vi "PPMS Interface_v230630.vi"() -> ()   [LabVIEW 2020]
panel:
  out "AC Flag":bool caption="AC Current"
  in  "Filetype":u16(ring)=2 items=[".xlsx", ".txt", ".csv"]
  out "Wait Done":dbl=10.0
  in  "Measurement setup tabs":enum32{"DC Setup", "AC Setup", "DC Delta Mode"}(tab)=enum."AC Setup"
  in  "DC Pulse":bool=TRUE caption="Current Pulsing"
  in  "Channel 2":bool=TRUE
  in  "Channel 1":bool
  in  "Current Amplitude":string="5e-4"
  in  "Time Period (s)":string="3"
  in  "Tpad(ms)":i32=200
  in  "Voltmeter Range (V)":string="0.01"
  in  "NPLC":string="1"
  in  "Voltmeter Buffer Size":string="62"
  in  "Voltmeter 2 Address":string="7"
  in  "Voltmeter 1 Address":string="8"
  in  "6221 Address":string="12"
  in  "Configure DC System":bool
  in  "6221 Address 2":string="12" caption="6221 Address"
  in  "Current Amplitude 2":string="100e-6" caption="Current \nAmplitude"
  in  "Ch2 Enable":bool=TRUE
  in  "Ch1 Enable":bool=TRUE
  in  "Buffer Data":enum16{"X", "XY", "RT", "XYRT"}(ring)=enum."RT"
  in  "Rate decimation":i32=2
  in  "SR860 Ch2 Address":string="5"
  in  "SR860 Ch1 Address":string="4"
  in  "Frequency":string="1711"
  in  "Filter BW":T1(ring)=enum."100ms"
  in  "Ch1 Harmonic":T2(ring)
  in  "Buffer Size (kB)":i32=2
  in  "Configure AC System":bool
  in  "Buffer Offset (kb)":string="0"
  in  "Ch2 Harmonic":T2(ring)=enum."2nd Harmonic"
  in  "Measurement \nSetup":u16(ring) items=["DC Setup", "AC Setup", "DC Delta Mode"]
  in  "Measure Device":bool caption="Measure \nDevice"
  in  "Y-axis":u16(ring)=6 items=["Serial Number", "Time Elapsed (s)", "Temperature (K)", "Field (Oe)", "Theta (degree)", "Current excitation (A)", "Resistance 1 (ohm)", "STD 1 (ohm)", "Resistance 2 (ohm)", "STD 2 (ohm)"]
  in  "X-axis":u16(ring)=3 items=["Serial Number", "Time Elapsed (s)", "Temperature (K)", "Field (Oe)", "Theta (degree)", "Current excitation (A)", "Resistance 1 (ohm)", "STD 1 (ohm)", "Resistance 2 (ohm)", "STD 2 (ohm)"]
  out "XY Graph":cluster{"Data array":dbl[], "Data array":dbl[]}(graph)={"Data array"=[1000.1076049804688, 1000.095458984375, 1000.1318969726562, 999.822021484375, 916.6700439453125, 830.8634643554688, 742.8192749023438, 654.9420776367188, 567.0899047851562, 479.1545104980469, 392.864013671875, 304.93212890625, 216.95523071289062, 129.0848846435547, 41.132198333740234, -44.77364730834961, -132.77415466308594, -218.81509399414062, -306.63739013671875, -394.50677490234375, -482.4195251464844, -570.4457397460938, -658.3638305664062, -744.2162475585938, -832.0615234375, -920.28857421875, -999.9136352539062, -999.8893432617188, -999.877197265625, -966.5936279296875, -880.3653564453125, -790.4647827148438, -704.466064453125, -616.628173828125, -528.7174682617188, -442.6363525390625, -352.7901916503906, -266.7317810058594, -178.9671173095703, -91.0753402709961, -3.042452096939087, 84.87220001220703, 170.94114685058594, 258.7779235839844, 346.6785583496094, 434.949462890625, 520.9051513671875, 608.9139404296875, 696.776611328125, 782.679931640625, 870.5813598632812, 958.4483642578125, 1000.1197509765625, 1000.095458984375], "Data array"=[2.0974435134090905, 2.0958316086363635, 2.0992071125, 2.0990977595454545, 2.107740888863636, 2.1053484827272726, 2.1082263649999997, 2.1037182222727275, 2.083242016590909, 2.081601890227273, 2.0829138438636363, 2.0798880874999996, 2.0791002761363635, 2.0677500127272728, 1.8619974204545455, 1.1222847387045454, 0.8201078938409091, 0.7255154414090907, 0.6976336516363636, 0.7003691852045455, 0.6927557248181818, 0.7014058921818181, 0.6990065759090907, 0.7079667083181819, 0.7010926857727272, 0.6957325292954544, 0.6955325533636365, 0.697872530181818, 0.711508848840909, 0.7229268473181818, 0.7067185125454545, 0.6959014081136364, 0.6962725788181818, 0.7031570712499998, 0.6892584726363638, 0.6798120112272727, 0.6948854190227274, 0.70866324875, 0.7220332009318181, 0.7281562234318182, 1.006325211, 1.7135642684090908, 1.949954792045455, 2.0590681531818182, 2.084260665, 2.087814913863636, 2.0882882709090906, 2.090093333181818, 2.0964560554545457, 2.1017757368181815, 2.103902046363636, 2.0958079104545453, 2.1060686974999996, 2.0965902061363635]}
  out "WAIT delay(s)":u32=10
  out "Data array":dbl[][](array[numeric])=[[1.0, 4.4622015953063965, 299.982421875, 1000.1076049804688, -0.00037384033203125, 0.0001, 2.0974435134090905, 0.003970427238917819, 0.023133111600000002, 0.00015789614384998], [2.0, 8.857791900634766, 299.9828186035156, 1000.095458984375, -0.00037384033203125, 0.0001, 2.0958316086363635, 0.005717710280839478, 0.023133111600000002, 0.00015789614384998], [3.0, 13.236927509307861, 299.9828186035156, 1000.1318969726562, -0.00037384033203125, 0.0001, 2.0992071125, 0.006189541986117072, 0.023133111600000002, 0.00015789614384998], [4.0, 17.593226432800293, 299.98480224609375, 999.822021484375, -0.00037384033203125, 0.0001, 2.0990977595454545, 0.003912224013200419, 0.023133111600000002, 0.00015789614384998], [5.0, 21.948697090148926, 299.9840087890625, 916.6700439453125, -0.00037384033203125, 0.0001, 2.107740888863636, 0.005090003201604339, 0.023133111600000002, 0.00015789614384998], [6.0, 26.332980155944824, 299.98516845703125, 830.8634643554688, -0.00037384033203125, 0.0001, 2.1053484827272726, 0.005739735103255567, 0.023133111600000002, 0.00015789614384998], [7.0, 30.68852186203003, 299.985595703125, 742.8192749023438, -0.00037384033203125, 0.0001, 2.1082263649999997, 0.005571697815375255, 0.023133111600000002, 0.00015789614384998], [8.0, 35.09347057342529, 299.98638916015625, 654.9420776367188, -0.00037384033203125, 0.0001, 2.1037182222727275, 0.00788260633201801, 0.023133111600000002, 0.00015789614384998], [9.0, 39.4463529586792, 299.98480224609375, 567.0899047851562, -0.00037384033203125, 0.0001, 2.083242016590909, 0.006414237562318937, 0.023133111600000002, 0.00015789614384998], [10.0, 43.830984115600586, 299.9861755371094, 479.1545104980469, -0.00037384033203125, 0.0001, 2.081601890227273, 0.005074439315863804, 0.023133111600000002, 0.00015789614384998], [11.0, 48.21513843536377, 299.98516845703125, 392.864013671875, -0.00037384033203125, 0.0001, 2.0829138438636363, 0.0047092558667783495, 0.023133111600000002, 0.00015789614384998], [12.0, 52.58274984359741, 299.9877624511719, 304.93212890625, -0.00037384033203125, 0.0001, 2.0798880874999996, 0.007156650519378263, 0.023133111600000002, 0.00015789614384998], [13.0, 56.942962646484375, 299.9867858886719, 216.95523071289062, -0.00037384033203125, 0.0001, 2.0791002761363635, 0.006338073258755396, 0.023133111600000002, 0.00015789614384998], [14.0, 61.33445596694946, 299.9844055175781, 129.0848846435547, -0.00037384033203125, 0.0001, 2.0677500127272728, 0.004479419760797201, 0.023133111600000002, 0.00015789614384998], [15.0, 65.69865989685059, 299.98516845703125, 41.132198333740234, -0.00037384033203125, 0.0001, 1.8619974204545455, 0.04372637509011968, 0.023133111600000002, 0.00015789614384998], [16.0, 70.06871700286865, 299.985595703125, -44.77364730834961, -0.00037384033203125, 0.0001, 1.1222847387045454, 0.04141744482498131, 0.023133111600000002, 0.00015789614384998], [17.0, 74.4264874458313, 299.98516845703125, -132.77415466308594, -0.00037384033203125, 0.0001, 0.8201078938409091, 0.012918566246848149, 0.023133111600000002, 0.00015789614384998], [18.0, 78.80255699157715, 299.985595703125, -218.81509399414062, -0.00037384033203125, 0.0001, 0.7255154414090907, 0.013867678751370198, 0.023133111600000002, 0.00015789614384998], [19.0, 83.20550107955933, 299.985595703125, -306.63739013671875, -0.00037384033203125, 0.0001, 0.6976336516363636, 0.005727042126808915, 0.023133111600000002, 0.00015789614384998], [20.0, 87.57900810241699, 299.9859619140625, -394.50677490234375, -0.00037384033203125, 0.0001, 0.7003691852045455, 0.006164392957730509, 0.023133111600000002, 0.00015789614384998], [21.0, 91.95004034042358, 299.98577880859375, -482.4195251464844, -0.00037384033203125, 0.0001, 0.6927557248181818, 0.005210320909525348, 0.023133111600000002, 0.00015789614384998], [22.0, 96.33998107910156, 299.9861755371094, -570.4457397460938, -0.00037384033203125, 0.0001, 0.7014058921818181, 0.004608349946130019, 0.023133111600000002, 0.00015789614384998], [23.0, 100.71973752975464, 299.98577880859375, -658.3638305664062, -0.00037384033203125, 0.0001, 0.6990065759090907, 0.003365288674988466, 0.023133111600000002, 0.00015789614384998], [24.0, 105.0504822731018, 299.98638916015625, -744.2162475585938, -0.00037384033203125, 0.0001, 0.7079667083181819, 0.006059950157953656, 0.023133111600000002, 0.00015789614384998], [25.0, 109.43017148971558, 299.9879455566406, -832.0615234375, -0.00037384033203125, 0.0001, 0.7010926857727272, 0.006067166646240939, 0.023133111600000002, 0.00015789614384998], [26.0, 113.79940557479858, 299.9875793457031, -920.28857421875, -0.00037384033203125, 0.0001, 0.6957325292954544, 0.005627155853698697, 0.023133111600000002, 0.00015789614384998], [27.0, 118.25392484664917, 299.9867858886719, -999.9136352539062, -0.00037384033203125, 0.0001, 0.6955325533636365, 0.00707814850177566, 0.023133111600000002, 0.00015789614384998], [28.0, 122.64683437347412, 299.985595703125, -999.8893432617188, -0.00037384033203125, 0.0001, 0.697872530181818, 0.004908374987900224, 0.023133111600000002, 0.00015789614384998], [29.0, 127.02530670166016, 299.9861755371094, -999.877197265625, -0.00037384033203125, 0.0001, 0.711508848840909, 0.004892085657814586, 0.023133111600000002, 0.00015789614384998], [30.0, 131.39422178268433, 299.98516845703125, -966.5936279296875, -0.00037384033203125, 0.0001, 0.7229268473181818, 0.0044813852811875655, 0.023133111600000002, 0.00015789614384998], [31.0, 135.83348321914673, 299.9867858886719, -880.3653564453125, -0.00037384033203125, 0.0001, 0.7067185125454545, 0.004279656852638706, 0.023133111600000002, 0.00015789614384998], [32.0, 140.21209907531738, 299.98516845703125, -790.4647827148438, -0.00037384033203125, 0.0001, 0.6959014081136364, 0.005017213765156999, 0.023133111600000002, 0.00015789614384998], [33.0, 144.59554243087769, 299.98638916015625, -704.466064453125, -0.00037384033203125, 0.0001, 0.6962725788181818, 0.007024556533565583, 0.023133111600000002, 0.00015789614384998], [34.0, 148.9465184211731, 299.9861755371094, -616.628173828125, -0.00037384033203125, 0.0001, 0.7031570712499998, 0.006011419658937474, 0.023133111600000002, 0.00015789614384998], [35.0, 153.31742238998413, 299.9883728027344, -528.7174682617188, -0.00037384033203125, 0.0001, 0.6892584726363638, 0.0056657125166453695, 0.023133111600000002, 0.00015789614384998], [36.0, 157.72580194473267, 299.9879455566406, -442.6363525390625, -0.00037384033203125, 0.0001, 0.6798120112272727, 0.006911608247074455, 0.023133111600000002, 0.00015789614384998], [37.0, 162.09323120117188, 299.98895263671875, -352.7901916503906, -0.00037384033203125, 0.0001, 0.6948854190227274, 0.005234077839025774, 0.023133111600000002, 0.00015789614384998], [38.0, 166.4765763282776, 299.9881591796875, -266.7317810058594, -0.00037384033203125, 0.0001, 0.70866324875, 0.004897465156522533, 0.023133111600000002, 0.00015789614384998], [39.0, 170.89887046813965, 299.9877624511719, -178.9671173095703, -0.00037384033203125, 0.0001, 0.7220332009318181, 0.004374043049098589, 0.023133111600000002, 0.00015789614384998], [40.0, 175.30081844329834, 299.98895263671875, -91.0753402709961, -0.00037384033203125, 0.0001, 0.7281562234318182, 0.004378933623760837, 0.023133111600000002, 0.00015789614384998], [41.0, 179.67326831817627, 299.9881591796875, -3.042452096939087, -0.00037384033203125, 0.0001, 1.006325211, 0.05479208135231416, 0.023133111600000002, 0.00015789614384998], [42.0, 184.02438020706177, 299.9891662597656, 84.87220001220703, -0.00037384033203125, 0.0001, 1.7135642684090908, 0.031492821331516825, 0.023133111600000002, 0.00015789614384998], [43.0, 188.40718173980713, 299.9934997558594, 170.94114685058594, -0.00037384033203125, 0.0001, 1.949954792045455, 0.005867722136927017, 0.023133111600000002, 0.00015789614384998], [44.0, 192.7843451499939, 299.992919921875, 258.7779235839844, -0.00037384033203125, 0.0001, 2.0590681531818182, 0.005339923736116385, 0.023133111600000002, 0.00015789614384998], [45.0, 197.14294481277466, 299.9942932128906, 346.6785583496094, -0.00037384033203125, 0.0001, 2.084260665, 0.006323898951825988, 0.023133111600000002, 0.00015789614384998], [46.0, 201.48842906951904, 299.9949035644531, 434.949462890625, -0.00037384033203125, 0.0001, 2.087814913863636, 0.005555079114947601, 0.023133111600000002, 0.00015789614384998], [47.0, 205.88358163833618, 299.9934997558594, 520.9051513671875, -0.00037384033203125, 0.0001, 2.0882882709090906, 0.006813247199825648, 0.023133111600000002, 0.00015789614384998], [48.0, 210.2482304573059, 299.9954833984375, 608.9139404296875, -0.00037384033203125, 0.0001, 2.090093333181818, 0.004951890810177865, 0.023133111600000002, 0.00015789614384998], [49.0, 214.59800720214844, 299.9941101074219, 696.776611328125, -0.00037384033203125, 0.0001, 2.0964560554545457, 0.005307616082520529, 0.023133111600000002, 0.00015789614384998], [50.0, 218.96898794174194, 299.99371337890625, 782.679931640625, -0.00037384033203125, 0.0001, 2.1017757368181815, 0.004526206790352821, 0.023133111600000002, 0.00015789614384998], [51.0, 223.39048957824707, 299.9945068359375, 870.5813598632812, -0.00037384033203125, 0.0001, 2.103902046363636, 0.005438989400576699, 0.023133111600000002, 0.00015789614384998], [52.0, 227.7996335029602, 299.99609375, 958.4483642578125, -0.00037384033203125, 0.0001, 2.0958079104545453, 0.005075665798007201, 0.023133111600000002, 0.00015789614384998], [53.0, 232.15194511413574, 299.9954833984375, 1000.1197509765625, -0.00037384033203125, 0.0001, 2.1060686974999996, 0.004951135996534981, 0.023133111600000002, 0.00015789614384998], [54.0, 236.54437589645386, 299.9950866699219, 1000.095458984375, -0.00037384033203125, 0.0001, 2.0965902061363635, 0.00573349701852997, 0.023133111600000002, 0.00015789614384998]]
  out "Time Elasped":dbl format="%#_13g"
  out "Serial Number":i32=55
  out "Current StartTime":timestamp=timestamp(3772308572.9414487 s since 1904-01-01)
  out "Current Filename":path=path "C:/Users/qmgmit/Desktop/Shivam/data/FGaT-WTe2/20230715_FGaT-WTe2_chip3_D1/test_sweep_0715_1929.csv"
  in  "Metadata":string="NbSe2 C1 6L\n50 uA, Rxx on Ch 2\n"
  out "SET Rate":dbl=20.0
  out "SET Setpoint":dbl=1000.0
  out "Current Line Number":i32=10
  out "Parameters":dbl[][](array[numeric])
  out "ENV VAR":string="MEASURE"
  out "Current Line":string="STOP MEASURE "
  out "Command":string="STOP"
  in  "Datafile Path":path=path "C:/Users/QDUser/Desktop/User Data/Shivam/NbSe2 devices/C1_6L/cooldown"
  out "Line Count":i32=10
  out "Array of commands":string[][](array[string])=[["## Field sweep to test device health"], ["NEWFILE test_sweep"], [""], ["START MEASURE"], ["WAIT MEASURE 10"], ["SET FIELD -1000 RATE 20"], ["WAIT FIELD 10"], ["SET FIELD 1000 RATE 20"], ["WAIT FIELD 10"], ["STOP MEASURE "]]
  out "Sequence File":string="## Field sweep to test device health\nNEWFILE test_sweep\n\nSTART MEASURE\nWAIT MEASURE 10\nSET FIELD -1000 RATE 20\nWAIT FIELD 10\nSET FIELD 1000 RATE 20\nWAIT FIELD 10\nSTOP MEASURE "
  in  "Sequence File":path=path "C:/Users/QDUser/Desktop/User Data/Shivam/NbSe2 devices/C1_6L/cooldown.lseq"
  out "STOP Flag":bool=TRUE
  out "Measure Blink":bool
  in  "Stop sequence":bool
  in  "Start Sequence":bool caption="Set Temperature"
  out "ExecSeq":bool caption="Executing Sequence"
  out "Measure Flag":bool caption="Measurement in progress"
  out "Field\nStatus":i32(ring)=4 items=["MagnetUnknown"=0, "StablePersistent"=1, "WarmingSwitch"=2, "CoolingSwitch"=3, "StableDriven"=4, "Iterating"=5, "Charging"=6, "Discharging"=7, "CurrentError"=8, "MagnetFailure"=15]
  out "Temperature\nStatus":i32(ring)=1 items=["TemperatureUnknown"=0, "Stable"=1, "Tracking"=2, "Near"=5, "Chasing"=6, "Filling"=7, "Standby"=10, "Disabled"=13, "ImpedanceNotFunction"=14, "TempFailure"=15]
  out "Chamber\nStatus":i32(ring)=1 items=["ChamberUnknown"=0, "PurgedAndSealed"=1, "VentedAndSealed"=2, "Sealed"=3, "Purging"=4, "Venting"=5, "PreHiVac"=6, "HighVac"=7, "PumpContinuous"=8, "VentContinuous"=9, "ChamberFailure"=15]
  out "Initialised":bool=TRUE
  in  "STOP Button":bool=TRUE
  in  "Set Chamber":bool caption="Set Temperature"
  in  "Set Position":bool caption="Set Temperature"
  in  "Set Field":bool caption="Set Temperature"
  in  "Set Temperature":bool
  in  "Chamber Setpoint":i32(ring)=5 caption="Chamber" items=["Seal", "PurgeAndSeal", "VentAndSeal", "PumpContinuous", "VentContinuous", "HighVacuum"]
  out "Theta":dbl=-0.00017547607421875 caption="Position"
  in  "Theta Setpoint":dbl caption="Theta (degrees)" min=-10.0 max=370.0
  out "Field":dbl=0.03621025010943413
  out "Temperature":dbl=299.9980773925781
  in  "Field Setpoint":dbl caption="Field (Oe)" min=-90000.0 max=90000.0
  in  "Temperature setpoint":dbl=10.0 caption="Temperature (K)" min=1.8 max=400.0
  in  "InstrumentType":i32(ring)=2 items=["PPMS", "VersaLab", "DynaCool", "SVSM", "OptiCool"]
  in  "Remote \nMode":bool
  in  "IP Address":string="10.29.163.8"
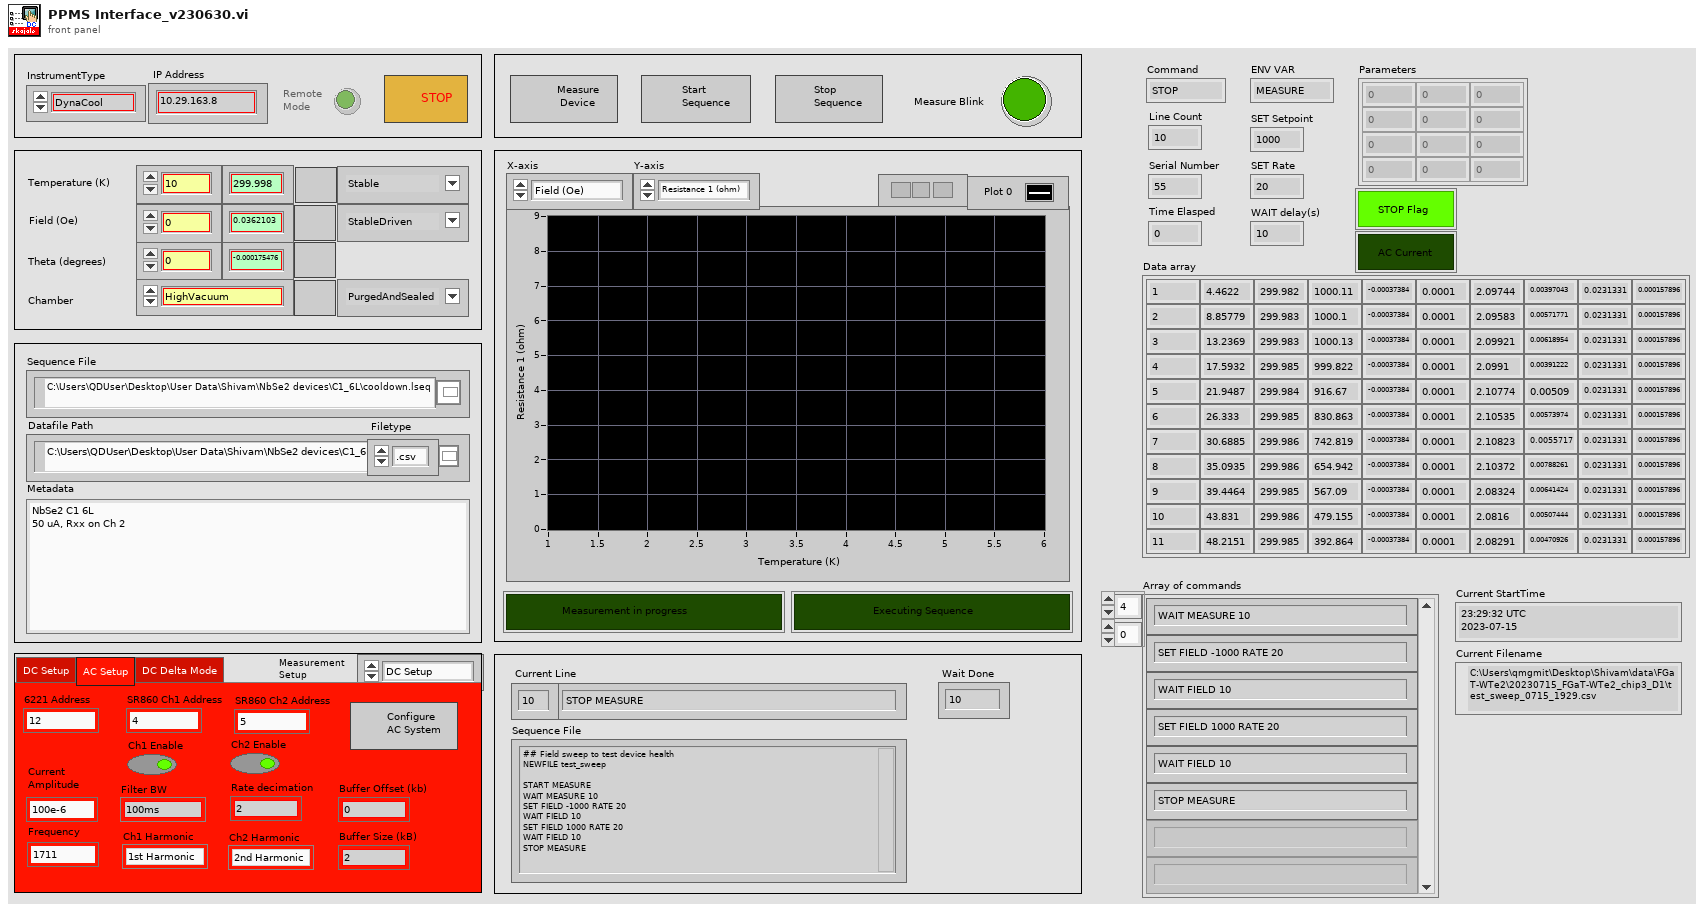
[diagram p1: front panel]
types:
  T1 = enum16{"1us", "3us", "10us", "30us", "100us", "300us", "1ms", "3ms", "10ms", "30ms", "100ms", "300ms", "1s"}
  T2 = enum16{"1st Harmonic", "2nd Harmonic", "3rd Harmonic"}
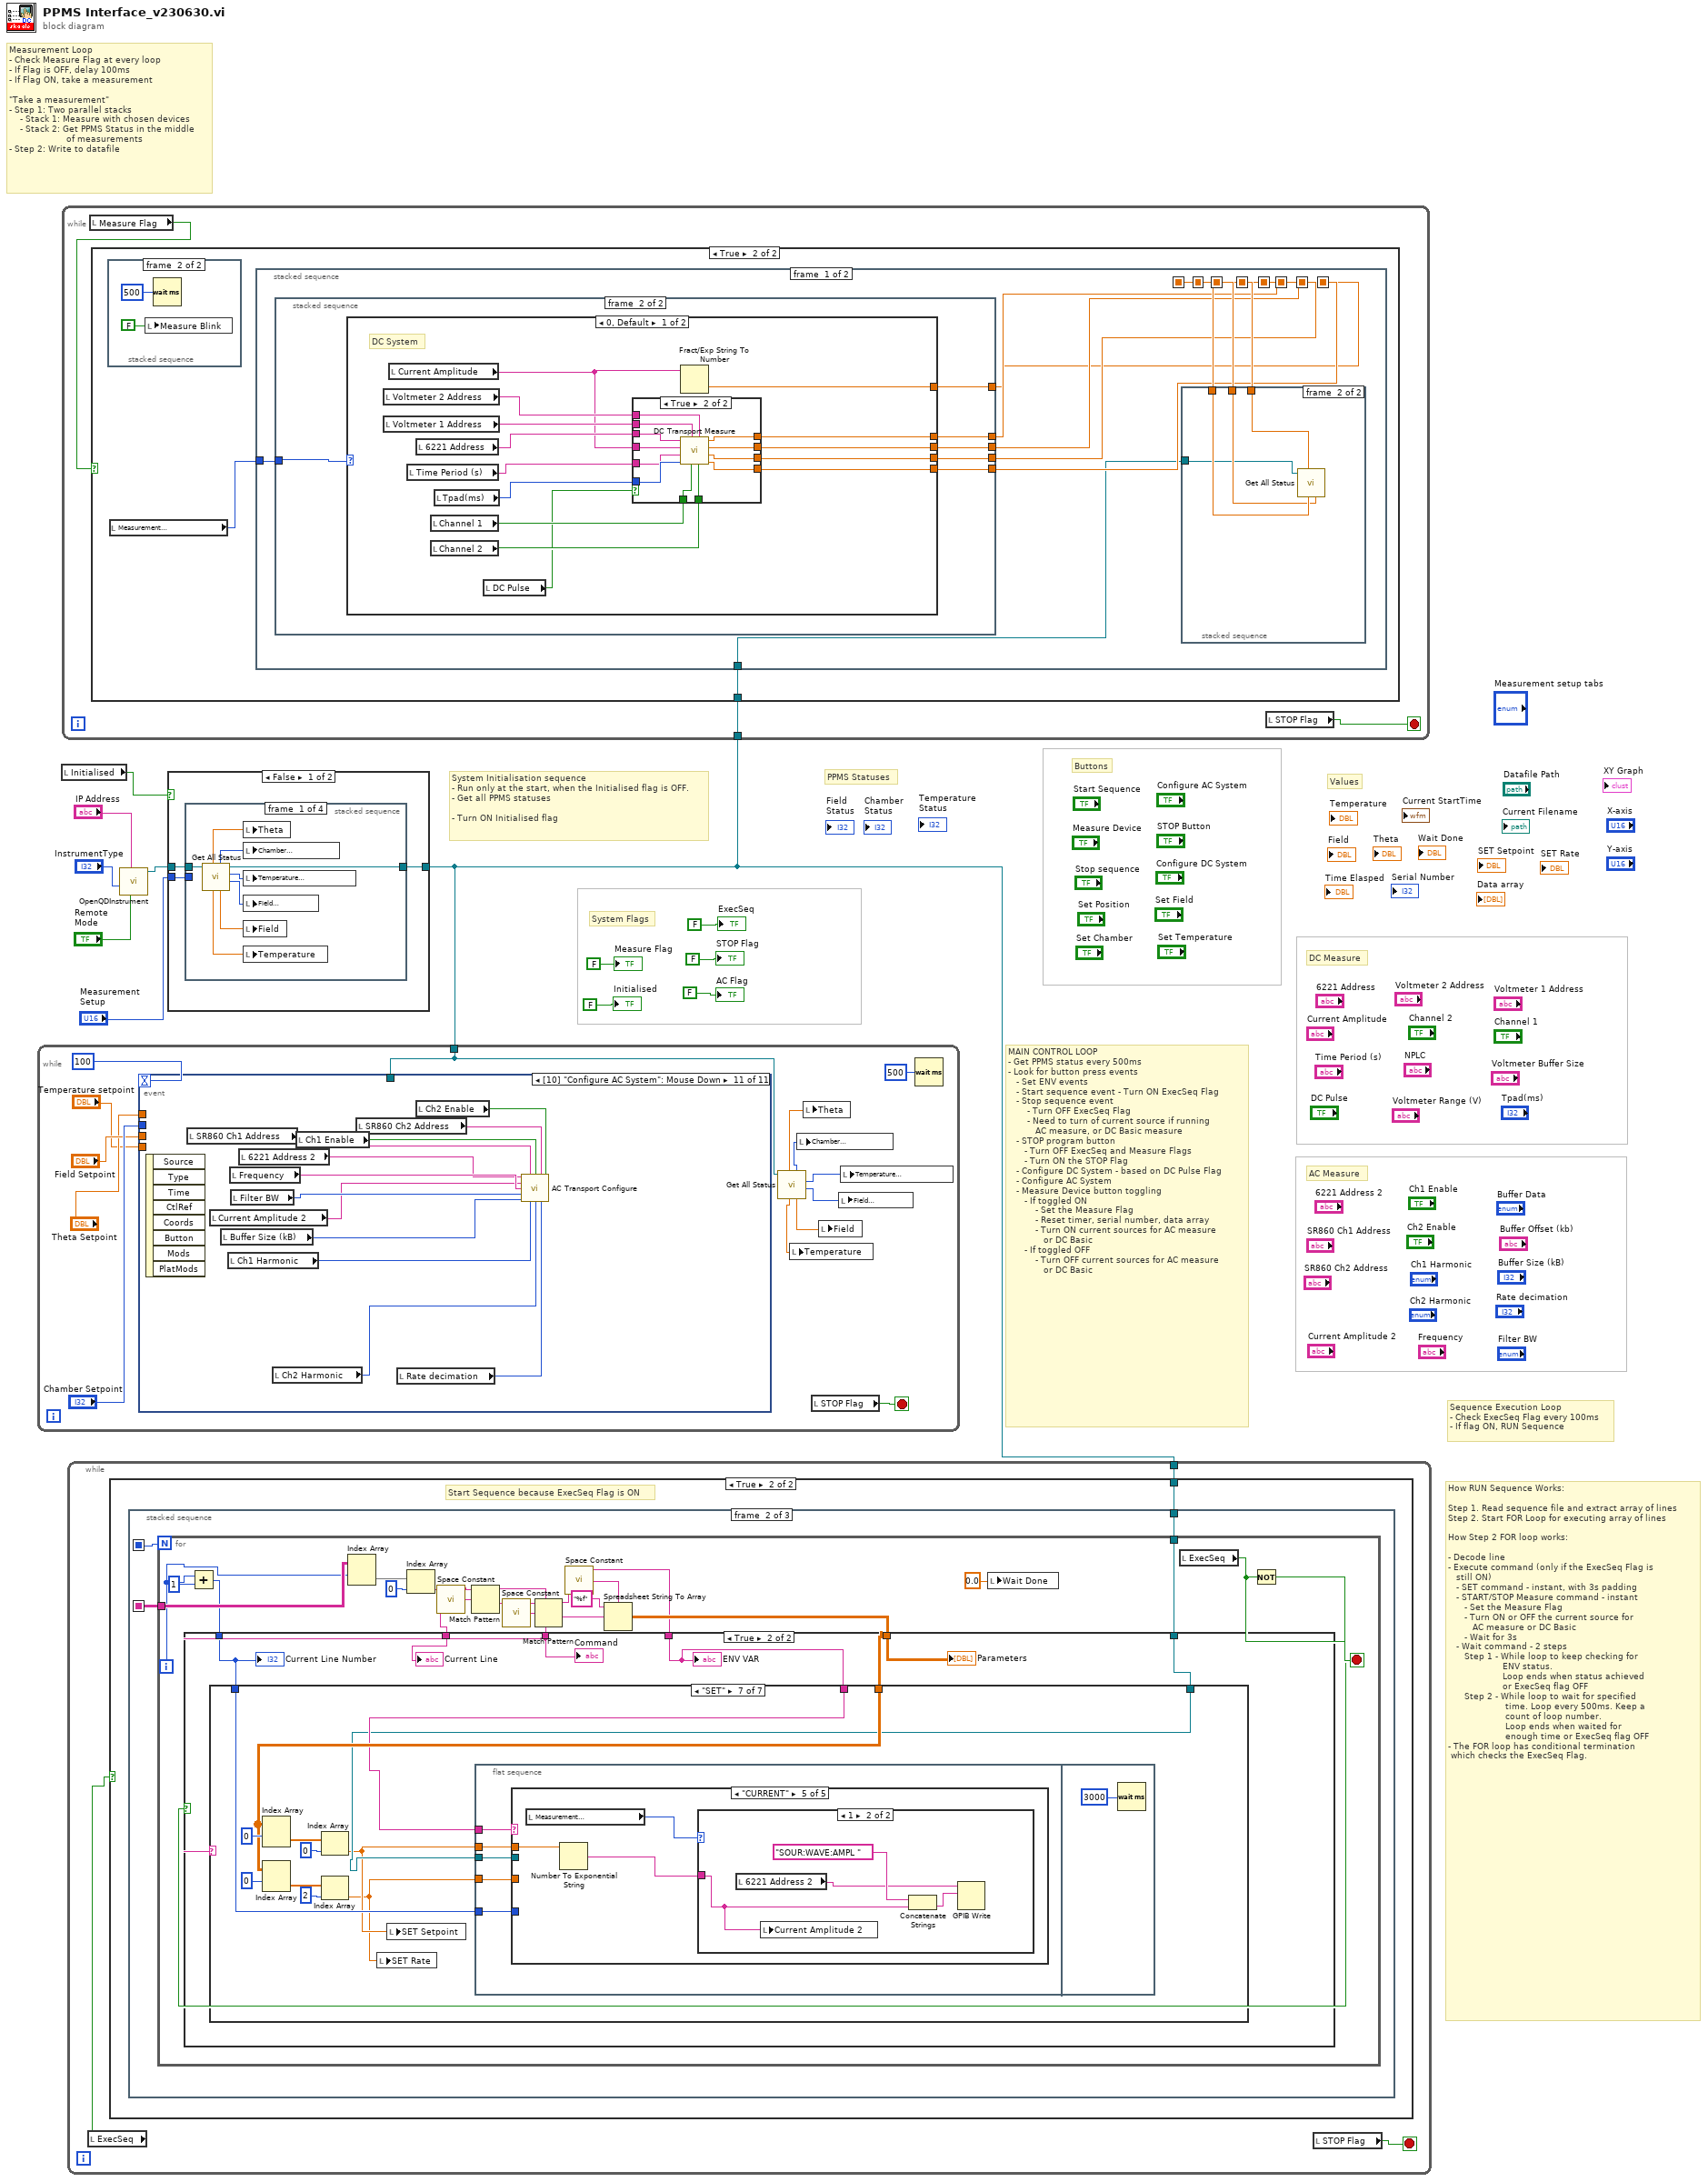
[diagram p0: block diagram]
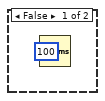
[diagram p2: hidden frame]
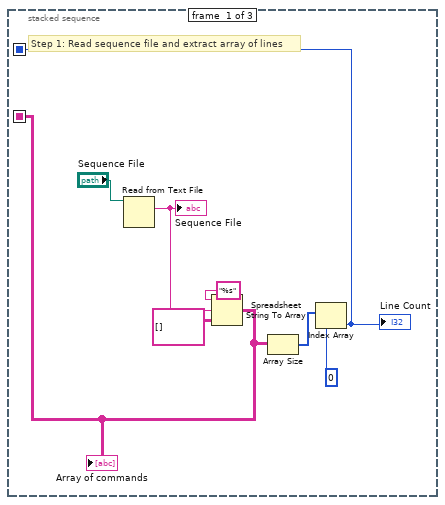
[diagram p3: hidden frame]
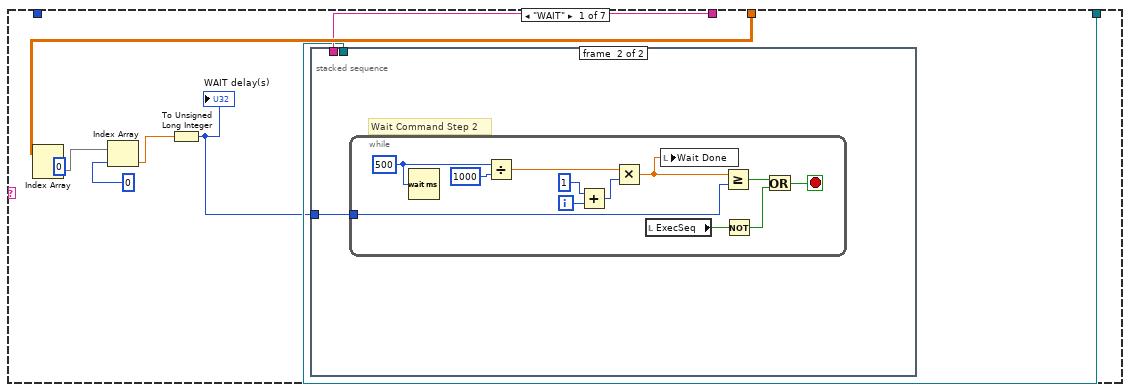
[diagram p5: hidden frame]
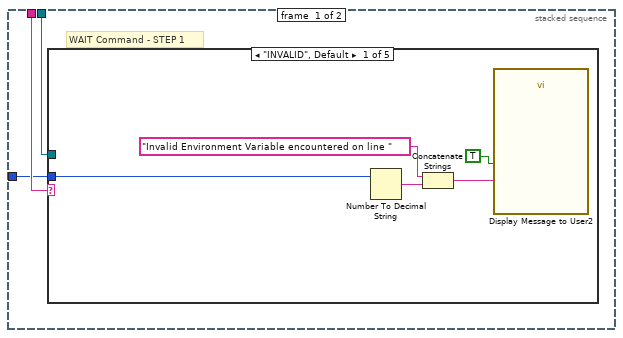
[diagram p6: hidden frame]
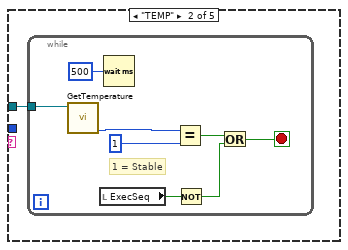
[diagram p7: hidden frame]
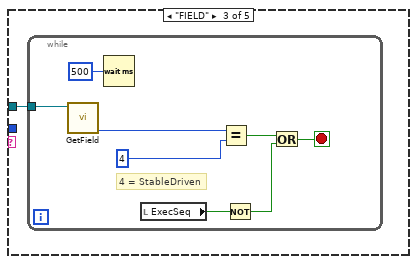
[diagram p8: hidden frame]
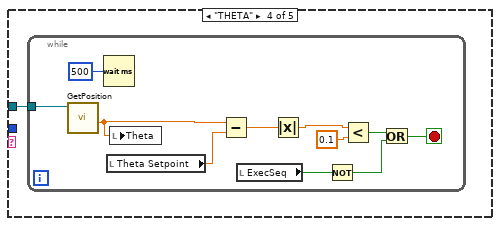
[diagram p9: hidden frame]
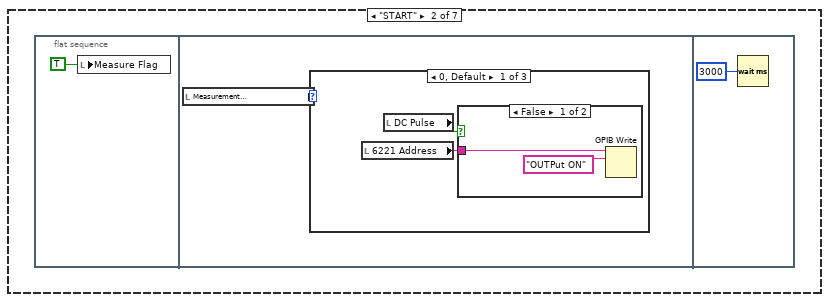
[diagram p11: hidden frame]
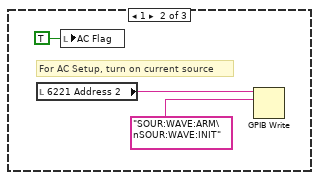
[diagram p13: hidden frame]
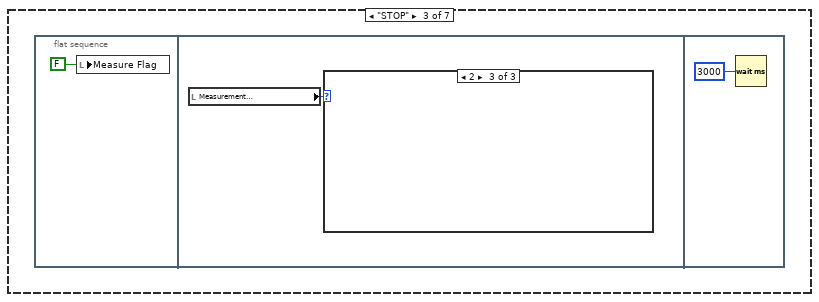
[diagram p15: hidden frame]
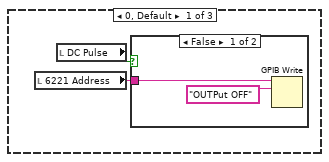
[diagram p16: hidden frame]
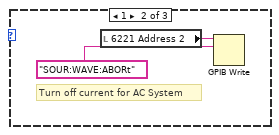
[diagram p18: hidden frame]
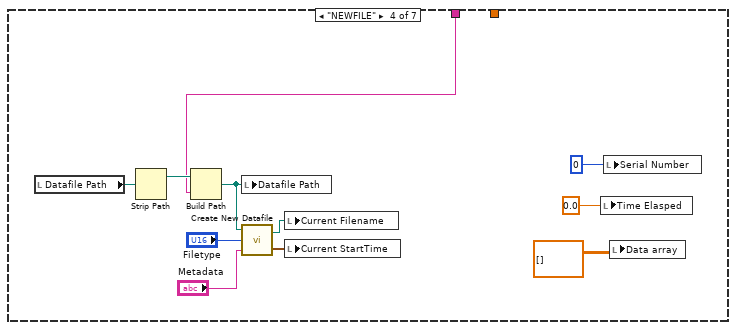
[diagram p19: hidden frame]
diagram:
  # "AC Measure"
  # "DC Measure"
  # "How RUN Sequence Works:\n\nStep 1. Read sequence file and extract array of lines \nStep 2. Start FOR Loop for executing array of lines\n\nHow Step 2 FOR loop works:\n\n- Decode line\n- Execute command (only if the ExecSeq Flag is \n   still ON)\n   - SET command - instant, with 3s padding\n   - START/STOP Measure command - instant\n      - Set the Measure Flag\n      - Turn ON or OFF the current source for \n         AC measure or DC Basic\n      - Wait for 3s\n   - Wait command - 2 steps\n      Step 1 - While loop to keep checking for\n                    ENV status.\n                    Loop ends when status achieved \n                    or ExecSeq flag OFF\n      Step 2 - While loop to wait for specified \n                     time. Loop every 500ms. Keep a \n                     count of loop number.\n                     Loop ends when waited for \n                     enough time or ExecSeq flag OFF\n- The FOR loop has conditional termination\n which checks the ExecSeq Flag."
  # "Sequence Execution Loop\n- Check ExecSeq Flag every 100ms\n- If flag ON, RUN Sequence"
  # "MAIN CONTROL LOOP\n- Get PPMS status every 500ms\n- Look for button press events\n   - Set ENV events\n   - Start sequence event - Turn ON ExecSeq Flag\n   - Stop sequence event \n       - Turn OFF ExecSeq Flag\n       - Need to turn of current source if running\n          AC measure, or DC Basic measure\n   - STOP program button \n      - Turn OFF ExecSeq and Measure Flags\n      - Turn ON the STOP Flag\n   - Configure DC System - based on DC Pulse Flag\n   - Configure AC System\n   - Measure Device button toggling\n      - If toggled ON \n          - Set the Measure Flag\n          - Reset timer, serial number, data array\n          - Turn ON current sources for AC measure \n             or DC Basic\n      - If toggled OFF\n          - Turn OFF current sources for AC measure \n             or DC Basic"
  # "System Flags"
  # "PPMS Statuses"
  # "Values"
  # "Buttons"
  # "System Initialisation sequence\n- Run only at the start, when the Initialised flag is OFF.\n- Get all PPMS statuses\n\n- Turn ON Initialised flag"
  # "Measurement Loop\n- Check Measure Flag at every loop\n- If Flag is OFF, delay 100ms\n- If Flag ON, take a measurement\n\n\"Take a measurement\"\n- Step 1: Two parallel stacks\n    - Stack 1: Measure with chosen devices\n    - Stack 2: Get PPMS Status in the middle\n                     of measurements\n- Step 2: Write to datafile"
  n1 = local read "Initialised"() -> (w8:bool)
  n2 = call "OpenQDInstrument.vi"("Remote"="Remote \nMode", "IP Address"="IP Address", "InstrumentType"="InstrumentType") -> ("Instrument Ref"=w7:refnum<k24>)  [unwired: 5 in, 1 out]
  n3 = case shown="False" w8 {
    tunnel: w7 -> [w15 w26]
    tunnel: [w14 w26] -> w3
    tunnel: "Measurement \nSetup" -> [w13 _]
    frame False {
      n4 = stacked-sequence {
        tunnel: w15 -> [w23 _ _ _]
        tunnel: [w17 _ _ _] -> w14
        tunnel: w13 -> [_ _ _ _]
        frame #0 {
          n5 = call "Get All Status.vi"("Instrument Ref In"=w23) -> ("Field\nStatus"=w20:i32, "Temperature\nStatus"=w21:i32, "Instrument Ref Out"=w17:refnum<k24>, "Field"=w18:dbl, "Chamber\nStatus"=w22:i32, "Temperature"=w19:dbl, "Position"=w16:dbl)  [unwired: 3 in, 1 out]
          n6 = local write "Theta"(w16) -> ()
          n7 = local write "Chamber\nStatus"(w22) -> ()
          n8 = local write "Temperature\nStatus"(w21) -> ()
          n9 = local write "Field\nStatus"(w20) -> ()
          n10 = local write "Field"(w18) -> ()
          n11 = local write "Temperature"(w19) -> ()
        }
        frame #1 {
          n12 = Wait (ms)(milliseconds to wait=u32 100) -> ()  [unwired: 1 out]
        }
        frame #2 {
        }
        frame #3 {
          n13 = local write "Initialised"(TRUE ("Initialised")) -> ()
        }
      }
    }
    frame True {
    }
  }
  n14 = while {
    tunnel: w3 -> [w31]
    stop <- w28 stop-if-true
    n15 = event shown="[10] \"Configure AC System\": Mouse Down" {
      selector: _ -> [_ _ _ _ _ _ _ _ _ _ _]
      dyn-events: _ -> [_ _ _ _ _ _ _ _ _ _ _]
      timeout: 100 -> [_ _ _ _ _ _ _ _ _ _ _]
      tunnel: "Chamber Setpoint" -> [_ _ w72 _ _ _ _ _ _ _ _]
      tunnel: w31 -> [_ _ w71 w76 w78 w82 _ _ _ _ _]
      tunnel: "Temperature setpoint" -> [_ _ _ w73 _ _ _ _ _ _ _]
      tunnel: "Field Setpoint" -> [_ _ _ _ w77 _ _ _ _ _ _]
      tunnel: "Theta Setpoint" -> [_ _ _ _ _ w81 _ _ _ _ _]
      event Timeout {
        # "Use timeout to update graph"
        n16 = event-data() -> ()  [unwired: 1 in, 3 out]
        n17 = local read "Data array"() -> (w48:dbl[][])
        n18 = property on="Y-axis" class="Ring (strict)"() -> ("RingText.Text"=w41:string)  [unwired: 2 in, 2 out]
        n19 = property on="X-axis" class="Ring (strict)"() -> ("RingText.Text"=w42:string)  [unwired: 2 in, 2 out]
        n20 = local read "Y-axis"() -> (w44:u16)
        n21 = local read "X-axis"() -> (w45:u16)
        n22 = Index Array(array=w48, index (col) #1=w45, index (col) #2=w44) -> (element #1=w47:dbl[], element #2=w46:dbl[])  [unwired: 2 in]
        n23 = Bundle("Data array"=w47, "Data array"=w46) -> (w43:cluster{"Data array":dbl[], "Data array":dbl[]})  [unwired: 1 in]
        n24 = property on="XY Graph" class="XYGraph (strict)"("XScale.NameLbl.Text"=w42, "YScale.NameLbl.Text"=w41) -> ()  [unwired: 2 in, 2 out]
        n25 = local write "XY Graph"(w43) -> ()
      }
      event "Measure Device": Value Change {
        n26 = event-data() -> ()  [unwired: 1 in, 6 out]
        n27 = local read "Measure Device"() -> (w49:bool)
        n28 = case shown="True" w49 {
          frame False {
            n29 = local read "Measurement \nSetup"() -> (w50:u16)
            n30 = case shown="0, Default" w50 {
              frame 0, Default {
                # "Turn off 6221 if DC Basic"
                n31 = local read "6221 Address"() -> (w51:string)
                n32 = local read "DC Pulse"() -> (w52:bool)
                n33 = case shown="False" w52 {
                  tunnel: w51 -> [w53 _]
                  frame False {
                    n34 = GPIB Write(0:w53, 1:"OUTPut OFF" ("data")) -> ()  [unwired: 3 in, 2 out]
                  }
                  frame True {
                  }
                }
              }
              frame 1 {
                # "Turn off 6221 for AC System"
                n35 = local read "6221 Address 2"() -> (w55:string)
                n36 = GPIB Write(0:w55, 1:"SOUR:WAVE:ABORt" ("data")) -> ()  [unwired: 3 in, 2 out]
              }
              frame 2 {
              }
            }
          }
          frame True {
            n37 = Get Date/Time In Seconds() -> (seconds since 1Jan1904=w58:timestamp)
            n38 = local write "Time Elasped"(0.0 ("Time Elasped")) -> ()
            n39 = local write "Serial Number"(0 ("Serial Number")) -> ()
            n40 = local read "Measurement \nSetup"() -> (w57:u16)
            n41 = local write "Current StartTime"(w58) -> ()
            n42 = local write "Data array"(dbl[][] [] ("Data array")) -> ()
            n43 = case shown="2" w57 {
              frame 0, Default {
                n44 = local read "6221 Address"() -> (w62:string)
                n45 = local read "DC Pulse"() -> (w63:bool)
                n46 = case shown="False" w63 {
                  tunnel: w62 -> [w65 _]
                  frame False {
                    n47 = Wait (ms)(milliseconds to wait=u32 1000) -> ()  [unwired: 1 out]
                    n48 = GPIB Write(0:w65, 1:"OUTPut ON" ("data")) -> ()  [unwired: 3 in, 2 out]
                  }
                  frame True {
                  }
                }
              }
              frame 1 {
                n49 = local read "6221 Address 2"() -> (w69:string)
                n50 = local write "AC Flag"(TRUE ("AC Flag")) -> ()
                n51 = Wait (ms)(milliseconds to wait=u32 1000) -> ()  [unwired: 1 out]
                n52 = GPIB Write(0:w69, 1:"SOUR:WAVE:ARM\nSOUR:WAVE:INIT" ("data")) -> ()  [unwired: 3 in, 2 out]
              }
              frame 2 {
              }
            }
          }
        }
        n53 = local write "Measure Flag"(w49) -> ()
      }
      event "Set Chamber": Mouse Down {
        n54 = event-data() -> ()  [unwired: 1 in, 8 out]
        n55 = call "SetChamber.vi"("Code"=w72, "Instrument Ref In"=w71) -> ()  [unwired: 1 in, 3 out]
      }
      event "Set Temperature": Mouse Down {
        w74 = 0 items=["FastSettle", "NoOvershoot"] ("Approach")
        n56 = event-data() -> ()  [unwired: 1 in, 8 out]
        n57 = call "SetTemperature.vi"("Approach"=w74, "Rate"=10.0, "Temperature"=w73, "Instrument Ref In"=w76) -> ()  [unwired: 3 in, 3 out]
      }
      event "Set Field": Mouse Down {
        n58 = event-data() -> ()  [unwired: 1 in, 8 out]
        n59 = call "SetField.vi"("Rate"=200.0, "Field"=w77, "Instrument Ref In"=w78) -> ()  [unwired: 4 in, 3 out]
      }
      event "Set Position": Mouse Down {
        n60 = event-data() -> ()  [unwired: 1 in, 8 out]
        n61 = call "SetPosition.vi"("Speed"=2.0, "Position"=w81, "Instrument Ref In"=w82) -> ()  [unwired: 4 in, 3 out]
      }
      event "Start Sequence": Mouse Down {
        n62 = event-data() -> ()  [unwired: 1 in, 8 out]
        n63 = local write "ExecSeq"(TRUE ("ExecSeq")) -> ()
      }
      event "Stop sequence": Mouse Down {
        w85 = FALSE ("ExecSeq")
        n64 = event-data() -> ()  [unwired: 1 in, 8 out]
        n65 = local read "Measurement \nSetup"() -> (w84:u16)
        n66 = local write "Measure Flag"(w85) -> ()
        n67 = local write "ExecSeq"(w85) -> ()
        n68 = case shown="0, Default" w84 {
          frame 0, Default {
            n69 = local read "6221 Address"() -> (w86:string)
            n70 = local read "DC Pulse"() -> (w87:bool)
            n71 = case shown="False" w87 {
              tunnel: w86 -> [w88 _]
              frame False {
                n72 = GPIB Write(0:w88, 1:"CURR OFF" ("data")) -> ()  [unwired: 3 in, 2 out]
              }
              frame True {
              }
            }
          }
          frame 1 {
            n73 = local read "6221 Address 2"() -> (w91:string)
            n74 = GPIB Write(0:w91, 1:"SOUR:WAVE:ABORt" ("data")) -> ()  [unwired: 3 in, 2 out]
          }
          frame 2 {
          }
        }
      }
      event "STOP Button": Mouse Down {
        n75 = event-data() -> ()  [unwired: 1 in, 8 out]
        n76 = stacked-sequence {
          frame #0 {
            w92 = FALSE ("Measure Flag")
            n77 = local write "ExecSeq"(w92) -> ()
            n78 = local write "Measure Flag"(w92) -> ()
          }
          frame #1 {
            n79 = Wait (ms)(milliseconds to wait=u32 1000) -> ()  [unwired: 1 out]
          }
          frame #2 {
            n80 = local write "STOP Flag"(TRUE ("STOP Flag")) -> ()
          }
        }
      }
      event "Configure DC System": Mouse Down {
        n81 = event-data() -> ()  [unwired: 1 in, 8 out]
        n82 = local read "Current Amplitude"() -> (w96:string)
        n83 = local read "Time Period (s)"() -> (w97:string)
        n84 = local read "6221 Address"() -> (w102:string)
        n85 = local read "Voltmeter Range (V)"() -> (w99:string)
        n86 = local read "NPLC"() -> (w98:string)
        n87 = local read "Voltmeter 1 Address"() -> (w103:string)
        n88 = local read "Voltmeter Buffer Size"() -> (w100:string)
        n89 = local read "Channel 2"() -> (w101:bool)
        n90 = local read "Voltmeter 2 Address"() -> (w104:string)
        n91 = local read "DC Pulse"() -> (w95:bool)
        n92 = local read "Channel 1"() -> (w105:bool)
        n93 = case shown="True" w95 {
          tunnel: w105 -> [w114 w124]
          tunnel: w104 -> [w113 w123]
          tunnel: w103 -> [w112 w122]
          tunnel: w102 -> [w111 w121]
          tunnel: w101 -> [w107 w120]
          tunnel: w100 -> [w106 w119]
          tunnel: w99 -> [w108 w118]
          tunnel: w98 -> [w109 w117]
          tunnel: w97 -> [_ w116]
          tunnel: w96 -> [w110 w115]
          frame False {
            n94 = call "DC Basic Configure.vi"("Channel 2"=w107, "Channel 1"=w114, "Voltmeter Buffer Size"=w106, "Voltmeter 2 Address"=w113, "Voltmeter Range (V)"=w108, "Voltmeter 1 Address"=w112, "NPLC"=w109, "Current Amplitude"=w110, "6221 Address"=w111) -> ()  [unwired: 3 in]
          }
          frame True {
            n95 = call "DC Transport Configure.vi"("Channel 2"=w120, "Channel 1"=w124, "Voltmeter Buffer Size"=w119, "Voltmeter 2 Address"=w123, "Voltmeter Range (V)"=w118, "Voltmeter 1 Address"=w122, "NPLC"=w117, "Time Period (s)"=w116, "Current Amplitude"=w115, "6221 Address"=w121) -> ()  [unwired: 2 in]
          }
        }
      }
      event "Configure AC System": Mouse Down {
        n96 = event-data() -> ()  [unwired: 1 in, 8 out]
        n97 = local read "SR860 Ch1 Address"() -> (w131:string)
        n98 = local read "Current Amplitude 2"() -> (w133:string)
        n99 = local read "Buffer Size (kB)"() -> (w127:i32)
        n100 = local read "Ch1 Harmonic"() -> (w126:T2)
        n101 = local read "Frequency"() -> (w134:string)
        n102 = local read "Filter BW"() -> (w135:T1)
        n103 = local read "6221 Address 2"() -> (w132:string)
        n104 = local read "Ch2 Harmonic"() -> (w125:T2)
        n105 = local read "Ch1 Enable"() -> (w130:bool)
        n106 = local read "SR860 Ch2 Address"() -> (w129:string)
        n107 = local read "Rate decimation"() -> (w136:i32)
        n108 = local read "Ch2 Enable"() -> (w128:bool)
        n109 = call "AC Transport Configure.vi"("6221 Address"=w132, "SR860 Ch1 Address"=w131, "Ch1 Enable"=w130, "SR860 Ch2 Address"=w129, "Ch2 Enable"=w128, "Current Amplitude"=w133, "Frequency"=w134, "Filter BW"=w135, "Buffer Size (kB)"=w127, "Ch1 Harmonic"=w126, "Ch2 Harmonic"=w125, "Rate decimation"=w136) -> ()  [unwired: 1 in, 3 out]
      }
    }
    n110 = call "Get All Status.vi"("Instrument Ref In"=w31) -> ("Field\nStatus"=w35:i32, "Temperature\nStatus"=w34:i32, "Field"=w37:dbl, "Chamber\nStatus"=w33:i32, "Temperature"=w36:dbl, "Position"=w30:dbl)  [unwired: 3 in, 2 out]
    n111 = local write "Temperature"(w36) -> ()
    n112 = local write "Chamber\nStatus"(w33) -> ()
    n113 = local write "Theta"(w30) -> ()
    n114 = local read "STOP Flag"() -> (w28:bool)
    n115 = local write "Field"(w37) -> ()
    n116 = local write "Field\nStatus"(w35) -> ()
    n117 = local write "Temperature\nStatus"(w34) -> ()
    n118 = Wait (ms)(milliseconds to wait=u32 500) -> ()  [unwired: 1 out]
  }
  n119 = while {
    tunnel: w3 -> [w137]
    stop <- w138 stop-if-true
    n120 = local read "Measure Flag"() -> (w139:bool)
    n121 = case shown="True" w139 {
      tunnel: w137 -> [_ w142]
      frame False {
        n122 = Wait (ms)(milliseconds to wait=u32 100) -> ()  [unwired: 1 out]
      }
      frame True {
        n123 = stacked-sequence {
          frame #0 {
            n124 = Wait (ms)(milliseconds to wait=u32 500) -> ()  [unwired: 1 out]
            "Measure Blink" <- TRUE ("Initialised")
          }
          frame #1 {
            n125 = local write "Measure Blink"(FALSE ("Measure Blink")) -> ()
            n126 = Wait (ms)(milliseconds to wait=u32 500) -> ()  [unwired: 1 out]
          }
        }
        n127 = local read "Measurement \nSetup"() -> (w141:u16)
        n128 = stacked-sequence {
          seq-local: [w150 _] -> [_ w245]
          seq-local: [w147 _] -> [_ w242]
          seq-local: [w146 _] -> [_ w243]
          seq-local: [w151 _] -> [_ w246]
          seq-local: [w152 _] -> [_ w247]
          seq-local: [w145 _] -> [_ w244]
          seq-local: [w149 _] -> [_ w240]
          seq-local: [w148 _] -> [_ w241]
          tunnel: w142 -> [w144 _]
          tunnel: w141 -> [w143 _]
          frame #0 {
            n129 = stacked-sequence {
              tunnel: w143 -> [_ w176]
              tunnel: [_ w181] -> w149
              tunnel: [_ w180] -> w148
              tunnel: [_ w179] -> w147
              tunnel: [_ w178] -> w146
              tunnel: [_ w177] -> w145
              frame #0 {
                # "If the flag is ON,\nwe wait for 5s to allow\nthe lock-in and current \nsource to settle.\nThen we turn off the flag\nto not do this again.\nThen we proceed to \nmeasurements."
                # "AC Flag is turned ON if\n- AC Current source of turned ON - inside sequence or with \"Measure Device\" button"
                n130 = local read "AC Flag"() -> (w153:bool)
                n131 = case shown="False" w153 {
                  frame False {
                  }
                  frame True {
                    n132 = stacked-sequence {
                      seq-local: [_ w159 _ _] -> [_ _ w169 _]
                      seq-local: [_ w157 _ _] -> [_ _ w167 _]
                      seq-local: [_ w156 _ _] -> [_ _ w166 _]
                      seq-local: [_ w155 _ _] -> [_ _ w165 _]
                      frame #0 {
                        n133 = Wait (ms)(milliseconds to wait=u32 1000) -> ()  [unwired: 1 out]
                      }
                      frame #1 {
                        w158 = "ARNG;\nASCL;" ("data")
                        n134 = local read "SR860 Ch2 Address"() -> (w155:string)
                        n135 = local read "Ch2 Enable"() -> (w156:bool)
                        n136 = local read "Ch1 Enable"() -> (w157:bool)
                        n137 = local read "SR860 Ch1 Address"() -> (w159:string)
                        n138 = case shown="True" w156 {
                          tunnel: w158 -> [_ w162]
                          tunnel: w155 -> [_ w161]
                          frame False {
                          }
                          frame True {
                            n139 = GPIB Write(0:w161, 1:w162) -> ()  [unwired: 3 in, 2 out]
                          }
                        }
                        n140 = case shown="True" w157 {
                          tunnel: w158 -> [_ w164]
                          tunnel: w159 -> [_ w163]
                          frame False {
                          }
                          frame True {
                            n141 = GPIB Write(0:w163, 1:w164) -> ()  [unwired: 3 in, 2 out]
                          }
                        }
                        n142 = Wait (ms)(milliseconds to wait=u32 1500) -> ()  [unwired: 1 out]
                      }
                      frame #2 {
                        w168 = "APHS;" ("data")
                        n143 = case shown="True" w166 {
                          tunnel: w168 -> [_ w172]
                          tunnel: w165 -> [_ w171]
                          frame False {
                          }
                          frame True {
                            n144 = GPIB Write(0:w171, 1:w172) -> ()  [unwired: 3 in, 2 out]
                          }
                        }
                        n145 = case shown="True" w167 {
                          tunnel: w169 -> [_ w174]
                          tunnel: w168 -> [_ w173]
                          frame False {
                          }
                          frame True {
                            n146 = GPIB Write(0:w174, 1:w173) -> ()  [unwired: 3 in, 2 out]
                          }
                        }
                        n147 = Wait (ms)(milliseconds to wait=u32 3500) -> ()  [unwired: 1 out]
                      }
                      frame #3 {
                        n148 = local write "AC Flag"(FALSE ("AC Flag")) -> ()
                      }
                    }
                  }
                }
              }
              frame #1 {
                n149 = case shown="0, Default" w176 {
                  tunnel: [w195 w218] -> w181
                  tunnel: [w194 w219] -> w180
                  tunnel: [w193 w220] -> w179
                  tunnel: [w192 w221] -> w178
                  tunnel: [w183 w226] -> w177
                  frame 0, Default {
                    # "DC System"
                    n150 = local read "Voltmeter 2 Address"() -> (w185:string)
                    n151 = local read "Voltmeter 1 Address"() -> (w186:string)
                    n152 = local read "Current Amplitude"() -> (w184:string)
                    n153 = local read "Time Period (s)"() -> (w188:string)
                    n154 = local read "6221 Address"() -> (w187:string)
                    n155 = local read "Channel 1"() -> (w190:bool)
                    n156 = local read "Channel 2"() -> (w191:bool)
                    n157 = local read "Tpad(ms)"() -> (w189:i32)
                    n158 = local read "DC Pulse"() -> (w182:bool)
                    n159 = case shown="True" w182 {
                      tunnel: [w205 w217] -> w195
                      tunnel: [w204 w216] -> w194
                      tunnel: [w203 w215] -> w193
                      tunnel: [w202 w214] -> w192
                      tunnel: w191 -> [w196 w213]
                      tunnel: w190 -> [w197 w212]
                      tunnel: w189 -> [_ w211]
                      tunnel: w188 -> [w198 w210]
                      tunnel: w187 -> [_ w209]
                      tunnel: w186 -> [w200 w208]
                      tunnel: w185 -> [w201 w207]
                      tunnel: w184 -> [w199 w206]
                      frame False {
                        n160 = call "DC Basic Measure.vi"("Channel 2"=w196, "Voltmeter 2 Address"=w201, "Channel 1"=w197, "Voltmeter 1 Address"=w200, "Period (s)"=w198, "Amplitude (A)"=w199) -> ("STD 2"=w202:dbl, "Resistance 2"=w203:dbl, "STD 1"=w204:dbl, "Resistance 1"=w205:dbl)  [unwired: 2 in]
                      }
                      frame True {
                        n161 = call "DC Transport Measure.vi"("Channel 2"=w213, "Voltmeter 2 Address"=w207, "Channel 1"=w212, "Voltmeter 1 Address"=w208, "tpad"=w211, "Period (s)"=w210, "Amplitude (A)"=w206, "6221 Address"=w209) -> ("STD 2"=w214:dbl, "Resistance 2"=w215:dbl, "STD 1"=w216:dbl, "Resistance 1"=w217:dbl)
                      }
                    }
                    n162 = Fract/Exp String To Number(string=w184) -> (number=w183:dbl)  [unwired: 3 in, 1 out]
                  }
                  frame 1 {
                    # "AC System"
                    n163 = local read "Buffer Offset (kb)"() -> (w230:string)
                    n164 = local read "Buffer Size (kB)"() -> (w229:i32)
                    n165 = local read "Ch1 Enable"() -> (w231:bool)
                    n166 = local read "Ch2 Enable"() -> (w228:bool)
                    n167 = local read "SR860 Ch1 Address"() -> (w232:string)
                    n168 = local read "SR860 Ch2 Address"() -> (w227:string)
                    n169 = local read "Current Amplitude 2"() -> (w233:string)
                    n170 = Fract/Exp String To Number(string=w233) -> (number=w226:dbl)  [unwired: 3 in, 1 out]
                    n171 = call "AC Transport Measure.vi"("SR860 Ch1 Address"=w232, "Ch1 Enable"=w231, "Buffer Offset (kb)"=w230, "Buffer Size (kb)"=w229, "Ch2 Enable"=w228, "SR860 Ch2 Address"=w227) -> ("R1 Mean"=w225:dbl, "R2 Mean"=w223:dbl, "R1 STD"=w224:dbl, "R2 STD"=w222:dbl)  [unwired: 6 in, 4 out]
                    n172 = Divide(x=w225, y=w226) -> (x/y=w218:dbl)
                    n173 = Divide(x=w224, y=w226) -> (x/y=w219:dbl)
                    n174 = Divide(x=w223, y=w226) -> (x/y=w220:dbl)
                    n175 = Divide(x=w222, y=w226) -> (x/y=w221:dbl)
                  }
                }
              }
            }
            n176 = stacked-sequence {
              tunnel: [_ w238] -> w152
              tunnel: [_ w237] -> w151
              tunnel: [_ w236] -> w150
              tunnel: w144 -> [_ w235]
              frame #0 {
                n177 = Wait (ms)(milliseconds to wait=u32 500) -> ()  [unwired: 1 out]
              }
              frame #1 {
                n178 = call "Get All Status.vi"("Instrument Ref In"=w235) -> ("Field"=w237:dbl, "Temperature"=w238:dbl, "Position"=w236:dbl)  [unwired: 3 in, 5 out]
              }
            }
          }
          frame #1 {
            # "Check measure flag before accumulating data as measure flag might've been turned off during the measurement period\nSuch a measurement is often garbage"
            n179 = local read "Serial Number"() -> (w252:i32)
            n180 = local read "Current StartTime"() -> (w248:timestamp)
            n181 = local read "Current Filename"() -> (w250:path)
            n182 = local read "Measure Flag"() -> (w239:bool)
            n183 = Add(x=w252, y=1) -> (x+y=w249:i32)
            n184 = local write "Serial Number"(w249) -> ()
            n185 = case shown="True" w239 {
              tunnel: w250 -> [_ w266]
              tunnel: w249 -> [_ w265]
              tunnel: w248 -> [_ w264]
              tunnel: w247 -> [_ w263]
              tunnel: w246 -> [_ w262]
              tunnel: w245 -> [_ w261]
              tunnel: w244 -> [_ w258]
              tunnel: w243 -> [_ w257]
              tunnel: w242 -> [_ w256]
              tunnel: w241 -> [_ w255]
              tunnel: w240 -> [_ w254]
              frame False {
              }
              frame True {
                n186 = local read "ExecSeq"() -> (w253:bool)
                n187 = case shown="True" w253 {
                  tunnel: w266 -> [_ w295]
                  tunnel: w265 -> [w283 w294]
                  tunnel: w264 -> [w282 w293]
                  tunnel: w263 -> [w280 w292]
                  tunnel: w262 -> [w279 w291]
                  tunnel: w261 -> [w278 w290]
                  tunnel: [w277 w289] -> w260
                  tunnel: w258 -> [w276 w288]
                  tunnel: w257 -> [w272 w287]
                  tunnel: w256 -> [w273 w286]
                  tunnel: w255 -> [w274 w285]
                  tunnel: w254 -> [w275 w284]
                  frame False {
                    n188 = Get Date/Time In Seconds() -> (seconds since 1Jan1904=w271:timestamp)
                    n189 = Subtract(x=w271, y=w282) -> (x-y=w281:dbl)
                    n190 = Build Array(w283, w281, w280, w279, w278, w276, w275, w274, w273, w272) -> (w277:dbl[])
                  }
                  frame True {
                    n191 = call "Create Datafile Entry.vi"("Serial Number"=w294, "Resistance 1"=w284, "STD 1"=w285, "File Name"=w295, "Start time"=w293, "Temperature"=w292, "Field"=w291, "Theta"=w290, "Resistance 2"=w286, "STD 2"=w287, "Current Level"=w288) -> ("Datapoint Array"=w289:dbl[])  [unwired: 3 in, 1 out]
                  }
                }
                n192 = Reshape Array(w260, 1 ("dimension size"), 10 ("dimension size")) -> (w259:dbl[][])
                n193 = local read "Data array"() -> (w268:dbl[][])
                n194 = Insert Into Array(array=w268, new element=w259) -> (w267:dbl[][])  [unwired: 2 in]
                n195 = local write "Data array"(w267) -> ()
              }
            }
          }
        }
      }
    }
    n196 = local read "STOP Flag"() -> (w138:bool)
  }
  n197 = while {
    tunnel: w3 -> [w300]
    stop <- w302 stop-if-true
    n198 = local read "ExecSeq"() -> (w301:bool)
    n199 = case shown="True" w301 {
      tunnel: w300 -> [_ w304]
      frame False {
        n200 = Wait (ms)(milliseconds to wait=u32 100) -> ()  [unwired: 1 out]
      }
      frame True {
        # "Start Sequence because ExecSeq Flag is ON"
        n201 = stacked-sequence {
          seq-local: [w306 _ _] -> [_ w315 _]
          seq-local: [w305 _ _] -> [_ w314 _]
          tunnel: w304 -> [_ w313 _]
          frame #0 {
            # "Step 1: Read sequence file and extract array of lines"
            n202 = Read from Text File(file (use dialog)="Sequence File") -> (text=w311:string)  [unwired: 3 in, 3 out]
            "Sequence File" <- w311
            n203 = Spreadsheet String To Array(format string="%s", spreadsheet string=w311, array type (2D Dbl)=string[][] []) -> (array=w305:string[][])  [unwired: 1 in]
            "Array of commands" <- w305
            n204 = Array Size(array=w305) -> (size(s)=w312:i32[])
            n205 = Index Array(array=w312, index=0) -> (element=w306:i32)
            "Line Count" <- w306
          }
          frame #1 {
            n206 = for {
              N: w315 -> [_]
              tunnel: w314 -> [w327]
              tunnel: w313 -> [w321]
              i -> [w318]
              stop <- w320 stop-if-true
              n207 = Add(x=w318, y=1) -> (x+y=w319:i32)
              n208 = Index Array(array=w327, index (row)=w318) -> (element=w326:string[])  [unwired: 1 in]
              n209 = Index Array(array=w326, index=0) -> (element=w325:string)
              n210 = call <vilib>:"Space Constant.vi"() -> ("String"=w335:string)
              n211 = Match Pattern(string=w325, regular expression=w335) -> (before substring=w324:string, after substring=w333:string)  [unwired: 1 in, 2 out]
              n212 = call <vilib>:"Space Constant.vi"() -> ("String"=w332:string)
              n213 = Match Pattern(string=w333, regular expression=w332) -> (before substring=w322:string, after substring=w330:string)  [unwired: 1 in, 2 out]
              n214 = call <vilib>:"Space Constant.vi"() -> ("String"=w329:string)
              n215 = Spreadsheet String To Array(delimiter (Tab)=w329, format string="%f", spreadsheet string=w330) -> (array=w323:dbl[][])  [unwired: 1 in]
              n216 = local write "Wait Done"(0.0 ("Wait Done")) -> ()
              n217 = local read "ExecSeq"() -> (w317:bool)
              n218 = case shown="True" w317 {
                tunnel: w325 -> [_ w341]
                tunnel: w324 -> [_ w340]
                tunnel: w323 -> [_ w339]
                tunnel: w322 -> [_ w338]
                tunnel: w321 -> [_ w337]
                tunnel: w319 -> [_ w336]
                frame False {
                }
                frame True {
                  n219 = case shown="\"SET\"" w340 {
                    tunnel: w339 -> [w345 _ _ _ _ _ w439]
                    tunnel: w338 -> [w344 _ _ w428 _ _ w436]
                    tunnel: w336 -> [_ _ _ _ _ _ w435]
                    tunnel: w337 -> [w343 _ _ _ _ _ w434]
                    frame "WAIT" {
                      n220 = Index Array(array=w345, index (row)=0) -> (element=w346:dbl[])  [unwired: 1 in]
                      n221 = Index Array(array=w346, index=0) -> (element=w347:dbl)
                      n222 = To Unsigned Long Integer(number=w347) -> (unsigned 32bit integer=w342:u32)
                      "WAIT delay(s)" <- w342
                      n223 = stacked-sequence {
                        tunnel: w344 -> [w352 _]
                        tunnel: w342 -> [w351 w388]
                        tunnel: w343 -> [w350 _]
                        frame #0 {
                          # "WAIT Command - STEP 1"
                          n224 = case shown="\"INVALID\", Default" w352 {
                            tunnel: w351 -> [w354 _ _ _ _]
                            tunnel: w350 -> [_ w358 w367 w376 _]
                            frame "INVALID", Default {
                              n225 = Number To Decimal String(number=w354) -> (decimal integer string=w355:string)  [unwired: 1 in]
                              n226 = Concatenate Strings("Invalid Environment Variable encountered on line " ("string"), w355) -> (w353:string)
                              n227 = call "Display Message to User2"("Enable"=TRUE, "Message"=w353) -> ()  [unwired: 8 in, 2 out]
                            }
                            frame "TEMP" {
                              n228 = while {
                                tunnel: w358 -> [w359]
                                stop <- w360 stop-if-true
                                # "1 = Stable"
                                n229 = call "GetTemperature.vi"("Instrument Ref In"=w359) -> ("Temperature\nStatus"=w364:i32)  [unwired: 4 in, 4 out]
                                n230 = local read "ExecSeq"() -> (w363:bool)
                                n231 = Wait (ms)(milliseconds to wait=u32 500) -> ()  [unwired: 1 out]
                                n232 = Equal?(x=w364, y=1) -> (x = y?=w362:bool)
                                n233 = Not(x=w363) -> (.not. x?=w361:bool)
                                n234 = Or(x=w362, y=w361) -> (x .or. y?=w360:bool)
                              }
                            }
                            frame "FIELD" {
                              n235 = while {
                                tunnel: w367 -> [w369]
                                stop <- w370 stop-if-true
                                # "4 = StableDriven"
                                n236 = call "GetField.vi"("Instrument Ref In"=w369) -> ("Field\nStatus"=w373:i32)  [unwired: 4 in, 4 out]
                                n237 = Wait (ms)(milliseconds to wait=u32 500) -> ()  [unwired: 1 out]
                                n238 = local read "ExecSeq"() -> (w372:bool)
                                n239 = Equal?(x=w373, y=4) -> (x = y?=w371:bool)
                                n240 = Not(x=w372) -> (.not. x?=w368:bool)
                                n241 = Or(x=w371, y=w368) -> (x .or. y?=w370:bool)
                              }
                            }
                            frame "THETA" {
                              n242 = while {
                                tunnel: w376 -> [w382]
                                stop <- w377 stop-if-true
                                n243 = call "GetPosition.vi"("Instrument Ref In"=w382) -> ("Position"=w386:dbl)  [unwired: 3 in, 3 out]
                                n244 = Wait (ms)(milliseconds to wait=u32 500) -> ()  [unwired: 1 out]
                                n245 = local read "Theta Setpoint"() -> (w381:dbl)
                                n246 = local write "Theta"(w386) -> ()
                                n247 = Subtract(x=w386, y=w381) -> (x-y=w385:dbl)
                                n248 = local read "ExecSeq"() -> (w380:bool)
                                n249 = Absolute Value(x=w385) -> (abs(x)=w384:dbl)
                                n250 = Not(x=w380) -> (.not. x?=w379:bool)
                                n251 = Less?(x=w384, y=0.1) -> (x < y?=w378:bool)
                                n252 = Or(x=w378, y=w379) -> (x .or. y?=w377:bool)
                              }
                            }
                            frame "MEASURE" {
                            }
                          }
                        }
                        frame #1 {
                          # "Wait Command Step 2"
                          n253 = while {
                            tunnel: w388 -> [w390]
                            i -> [w399]
                            stop <- w394 stop-if-true
                            w398 = u32 500 ("milliseconds to wait")
                            n254 = Wait (ms)(milliseconds to wait=w398) -> ()  [unwired: 1 out]
                            n255 = Divide(x=w398, y=u32 1000) -> (x/y=w396:dbl)
                            n256 = Add(x=1, y=w399) -> (x+y=w392:i32)
                            n257 = Multiply(x=w396, y=w392) -> (x*y=w389:dbl)
                            n258 = local read "ExecSeq"() -> (w400:bool)
                            n259 = local write "Wait Done"(w389) -> ()
                            n260 = Greater Or Equal?(x=w389, y=w390) -> (x >= y?=w395:bool)
                            n261 = Not(x=w400) -> (.not. x?=w393:bool)
                            n262 = Or(x=w395, y=w393) -> (x .or. y?=w394:bool)
                          }
                        }
                      }
                    }
                    frame "START" {
                      n263 = flat-sequence {
                        frame #0 {
                          n264 = local write "Measure Flag"(TRUE ("Measure Flag")) -> ()
                        }
                        frame #1 {
                          n265 = local read "Measurement \nSetup"() -> (w402:u16)
                          n266 = case shown="0, Default" w402 {
                            frame 0, Default {
                              n267 = local read "6221 Address"() -> (w403:string)
                              n268 = local read "DC Pulse"() -> (w404:bool)
                              n269 = case shown="False" w404 {
                                tunnel: w403 -> [w405 _]
                                frame False {
                                n270 = GPIB Write(0:w405, 1:"OUTPut ON" ("data")) -> ()  [unwired: 3 in, 2 out]
                                }
                                frame True {
                                }
                              }
                            }
                            frame 1 {
                              # "For AC Setup, turn on current source"
                              n271 = local read "6221 Address 2"() -> (w409:string)
                              n272 = local write "AC Flag"(TRUE ("AC Flag")) -> ()
                              n273 = GPIB Write(0:w409, 1:"SOUR:WAVE:ARM\nSOUR:WAVE:INIT" ("data")) -> ()  [unwired: 3 in, 2 out]
                            }
                            frame 2 {
                            }
                          }
                        }
                        frame #2 {
                          n274 = Wait (ms)(milliseconds to wait=u32 3000) -> ()  [unwired: 1 out]
                        }
                      }
                    }
                    frame "STOP" {
                      n275 = flat-sequence {
                        frame #0 {
                          n276 = local write "Measure Flag"(FALSE ("Measure Flag")) -> ()
                        }
                        frame #1 {
                          n277 = local read "Measurement \nSetup"() -> (w412:u16)
                          n278 = case shown="2" w412 {
                            frame 0, Default {
                              n279 = local read "6221 Address"() -> (w413:string)
                              n280 = local read "DC Pulse"() -> (w414:bool)
                              n281 = case shown="False" w414 {
                                tunnel: w413 -> [w415 _]
                                frame False {
                                n282 = GPIB Write(0:w415, 1:"OUTPut OFF" ("data")) -> ()  [unwired: 3 in, 2 out]
                                }
                                frame True {
                                }
                              }
                            }
                            frame 1 {
                              # "Turn off current for AC System"
                              n283 = local read "6221 Address 2"() -> (w417:string)
                              n284 = GPIB Write(0:w417, 1:"SOUR:WAVE:ABORt" ("data")) -> ()  [unwired: 3 in, 2 out]
                            }
                            frame 2 {
                            }
                          }
                        }
                        frame #2 {
                          n285 = Wait (ms)(milliseconds to wait=u32 3000) -> ()  [unwired: 1 out]
                        }
                      }
                    }
                    frame "NEWFILE" {
                      n286 = local read "Datafile Path"() -> (w430:path)
                      n287 = Strip Path(path=w430) -> (stripped path=w429:path)  [unwired: 1 out]
                      n288 = Build Path(base path=w429, name or relative path=w428) -> (appended path=w427:path)
                      n289 = local write "Datafile Path"(w427) -> ()
                      n290 = call "Create New Datafile.vi"("Metadata"="Metadata", "Filetype"="Filetype", "File Base"=w427) -> ("Start time"=w424:timestamp, "File name"=w425:path)
                      n291 = local write "Current Filename"(w425) -> ()
                      n292 = local write "Current StartTime"(w424) -> ()
                      n293 = local write "Time Elasped"(0.0 ("Time Elasped")) -> ()
                      n294 = local write "Serial Number"(0) -> ()
                      n295 = local write "Data array"(dbl[][] [] ("Data array")) -> ()
                    }
                    frame "#", Default {
                      # "Let go. This is considered a comment"
                    }
                    frame "" {
                      # "Blank line disregarded as a comment"
                    }
                    frame "SET" {
                      n296 = Index Array(array=w439, index (row)=0) -> (element=w438:dbl[])  [unwired: 1 in]
                      n297 = Index Array(array=w439, index (row)=0) -> (element=w437:dbl[])  [unwired: 1 in]
                      n298 = Index Array(array=w438, index=0) -> (element=w433:dbl)
                      n299 = Index Array(array=w437, index=2) -> (element=w432:dbl)
                      n300 = local write "SET Rate"(w432) -> ()
                      n301 = local write "SET Setpoint"(w433) -> ()
                      n302 = flat-sequence {
                        tunnel: w436 -> [w447]
                        tunnel: w435 -> [w446]
                        tunnel: w434 -> [w445]
                        tunnel: w433 -> [w444]
                        tunnel: w432 -> [w443]
                        frame #0 {
                          n303 = case shown="\"CURRENT\"" w447 {
                            tunnel: w446 -> [w448 _ _ _ _]
                            tunnel: w445 -> [_ w455 w458 w461 _]
                            tunnel: w444 -> [_ w453 w457 w460 w465]
                            tunnel: w443 -> [_ w454 w459 w462 _]
                            frame "INVALID", Default {
                              n304 = Number To Decimal String(number=w448) -> (decimal integer string=w450:string)  [unwired: 1 in]
                              n305 = Concatenate Strings("Invalid Environment Variable encountered on line " ("string"), w450) -> (w449:string)
                              n306 = call "Display Message to User"("Enable"=TRUE, "Message"=w449) -> ()  [unwired: 8 in, 2 out]
                            }
                            frame "TEMP" {
                              w456 = 0 items=["FastSettle", "NoOvershoot"] ("Approach")
                              n307 = call "SetTemperature.vi"("Approach"=w456, "Rate"=w454, "Temperature"=w453, "Instrument Ref In"=w455) -> ()  [unwired: 3 in, 3 out]
                              n308 = local write "Temperature setpoint"(w453) -> ()
                            }
                            frame "FIELD" {
                              n309 = call "SetField.vi"("Rate"=w459, "Field"=w457, "Instrument Ref In"=w458) -> ()  [unwired: 4 in, 3 out]
                              n310 = local write "Field Setpoint"(w457) -> ()
                            }
                            frame "THETA" {
                              n311 = local write "Theta Setpoint"(w460) -> ()
                              n312 = call "SetPosition.vi"("Speed"=w462, "Position"=w460, "Instrument Ref In"=w461) -> ()  [unwired: 4 in, 3 out]
                            }
                            frame "CURRENT" {
                              n313 = local read "Measurement \nSetup"() -> (w463:u16)
                              n314 = Number To Exponential String(number=w465) -> (E-format string=w464:string)  [unwired: 3 in]
                              n315 = case shown="1" w463 {
                                tunnel: w464 -> [w466 w477]
                                frame 0, Default {
                                n316 = local read "6221 Address"() -> (w468:string)
                                n317 = local write "Current Amplitude"(w466) -> ()
                                n318 = local read "DC Pulse"() -> (w467:bool)
                                n319 = case shown="True" w467 {
                                tunnel: w468 -> [w471 w474]
                                tunnel: w466 -> [w469 w475]
                                frame False {
                                n320 = Concatenate Strings("CURRent ", w469) -> (w470:string)
                                n321 = GPIB Write(0:w471, 1:w470) -> ()  [unwired: 3 in, 2 out]
                                }
                                frame True {
                                n322 = Concatenate Strings("SOUR:WAVE:AMPL " ("string"), w475) -> (w476:string)
                                n323 = GPIB Write(0:w474, 1:w476) -> ()  [unwired: 3 in, 2 out]
                                }
                                }
                                }
                                frame 1 {
                                n324 = local read "6221 Address 2"() -> (w478:string)
                                n325 = local write "Current Amplitude 2"(w477) -> ()
                                n326 = Concatenate Strings("SOUR:WAVE:AMPL " ("string"), w477) -> (w480:string)
                                n327 = GPIB Write(0:w478, 1:w480) -> ()  [unwired: 3 in, 2 out]
                                }
                              }
                            }
                          }
                        }
                        frame #1 {
                          n328 = Wait (ms)(milliseconds to wait=u32 3000) -> ()  [unwired: 1 out]
                        }
                      }
                    }
                  }
                  "Command" <- w340
                  "Current Line" <- w341
                  "ENV VAR" <- w338
                  "Parameters" <- w339
                  "Current Line Number" <- w336
                }
              }
              n329 = Not(x=w317) -> (.not. x?=w320:bool)
            }
          }
          frame #2 {
            n330 = local write "ExecSeq"(FALSE ("ExecSeq")) -> ()
          }
        }
      }
    }
    n331 = local read "STOP Flag"() -> (w302:bool)
  }
  "Initialised" <- FALSE ("Initialised")
  "Measure Flag" <- FALSE ("Measure Flag")
  "ExecSeq" <- FALSE ("Initialised")
  "STOP Flag" <- FALSE ("Initialised")
  "AC Flag" <- FALSE ("AC Current Flag")
